vi "VariantToPlainText (Standard).vi"(11 "Variant-formatted Value":variant) -> (3 "String-formatted Value":string)   [LabVIEW 2013, in "OpenSerializer.lvlib" / "Serializer.PlainText.lvclass"]
uses:
  Serializer.PlainText.lvclass
  <vilib>/LabVIEW Open Source Project/Data Manipulation/TypeDescriptor/TypeDescriptor_GetName.vi
  <vilib>/LabVIEW Open Source Project/Data Manipulation/TypeDescriptor/TypeDescriptor_GetType.vi
  <vilib>/LabVIEW Open Source Project/Data Manipulation/TypeDescriptor/TypeDescriptor_GetPString.vi
  <vilib>/LabVIEW Open Source Project/Data Manipulation/Conversions/Flattened nD-Array to Flattened 1D-Array.vi
  <vilib>/Utility/VariantDataType/VariantType.lvlib
  <vilib>/LabVIEW Open Source Project/Data Manipulation/TypeDescriptor/OpenDescriptor.lvlib
  <vilib>/LabVIEW Open Source Project/Data Manipulation/Variant/OpenVariant.lvlib
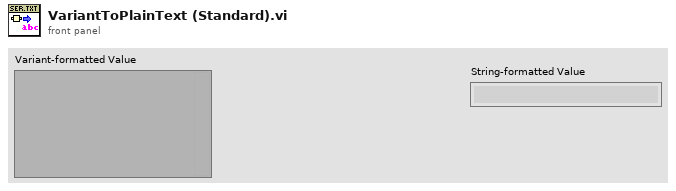
[diagram p1: front panel]
types:
  T1 = typedef "VariantType.lvlib/Type.ctl" = enum8{"Invalid Type", "Void", "I8", "I16", "I32", "I64", "U8", "U16", "U32", "U64", "Single Float", "Double Float", "Extended Float", "Single Complex", "Double Complex", "Extended Complex", "Enum U8", "Enum U16", "Enum U32", "Enum U64", "Single Float With Unit", "Double Float With Unit", "Extended Float With Unit", "Single Complex with Unit", "Double Complex with Unit", "Extended Complex with Unit", "Boolean", "String", "Path", "Picture", "Tag", "Array", "Cluster", "Variant", "LV Variant", "Waveform", "Timestamp", "Digital Waveform", "Digital Data", "ExpressData", "Refnum", "External Data", "VI", "Poly VI", "LabVIEW Class Instance", "Fixed Point"}
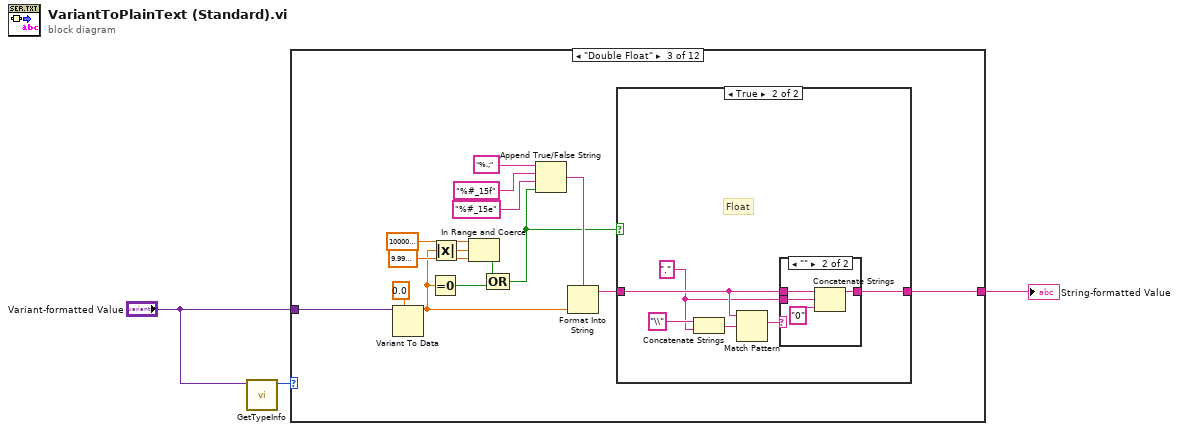
[diagram p0: block diagram]
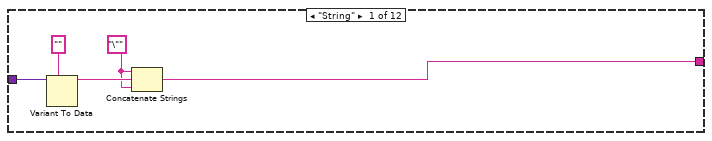
[diagram p2: hidden frame]
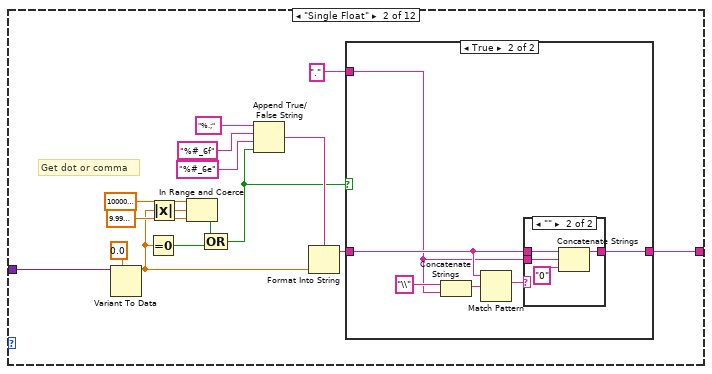
[diagram p3: hidden frame]
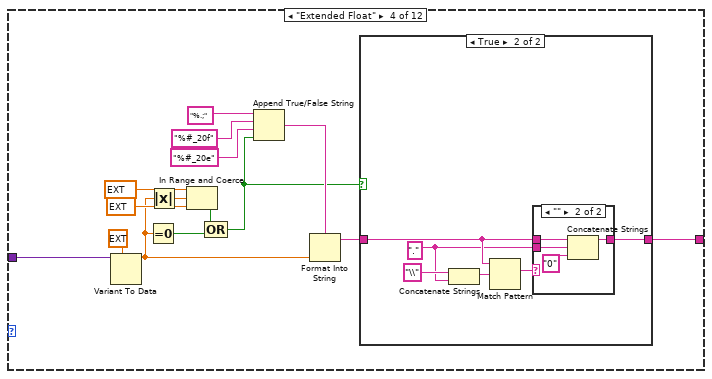
[diagram p8: hidden frame]
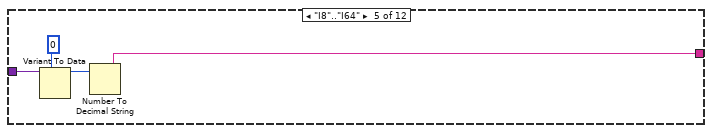
[diagram p11: hidden frame]
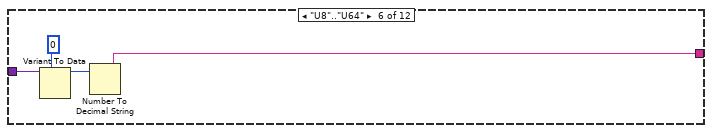
[diagram p12: hidden frame]
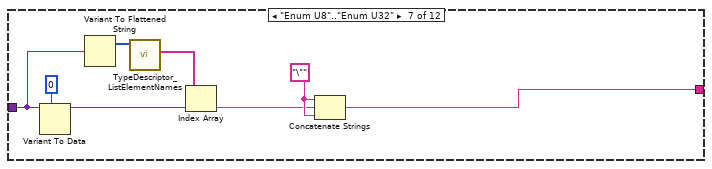
[diagram p13: hidden frame]
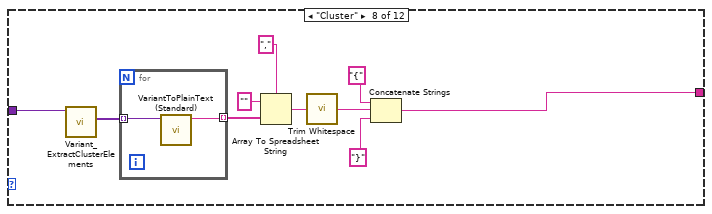
[diagram p14: hidden frame]
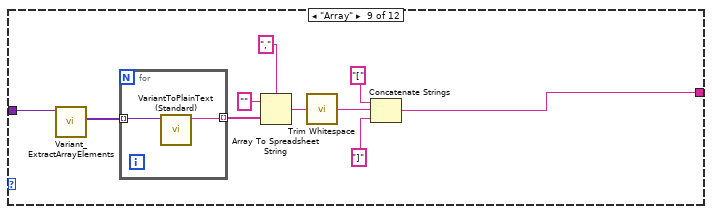
[diagram p15: hidden frame]
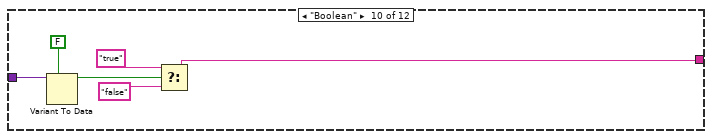
[diagram p16: hidden frame]
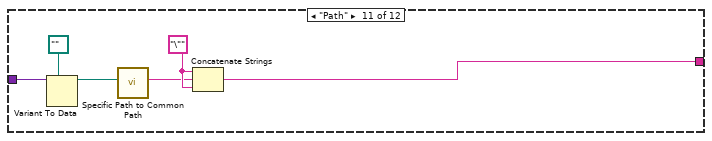
[diagram p17: hidden frame]
diagram:
  n1 = call <vilib>:"GetTypeInfo.vi"("Variant"="Variant-formatted Value") -> ("Type Enum"=w3:T1)  [unwired: 6 in, 4 out]
  n2 = case shown="\"Double Float\"" w3 {
    tunnel: "Variant-formatted Value" -> [w8 w18 w45 w72 w92 w96 w105 w113 w120 w136 w142 _]
    tunnel: [w5 w13 w40 w67 w91 w95 w99 w115 w127 w133 w139 _] -> w1
    frame "String" {
      w4 = "\"" ("Format String")
      n3 = Variant To Data(type="" ("Format String"), Variant=w8) -> (data=w6:string)  [unwired: 1 in, 1 out]
      n4 = Concatenate Strings(w4, w6, w4) -> (w5:string)
    }
    frame "Single Float" {
      # "Get dot or comma"
      n5 = Variant To Data(type=sgl 0.0, Variant=w18) -> (data=w15:sgl)  [unwired: 1 in, 1 out]
      n6 = Equal To 0?(x=w15) -> (x = 0?=w20:bool)
      n7 = Absolute Value(x=w15) -> (abs(x)=w21:sgl)
      n8 = In Range and Coerce(upper limit=sgl 1000000.0, x=w21, lower limit=sgl 0.0001 ("upper limit")) -> (In Range?=w19:bool)  [unwired: 1 out]
      n9 = Compound Arithmetic op=OR(w19, w20) -> (w11:bool)
      n10 = Append True/False String(1:w11, 2:"%#_6e" ("format string"), 3:"%#_6f" ("format string"), 4:"%.;" ("format string")) -> (0:w14:string)
      n11 = Format Into String(format string=w14, w15) -> (resulting string=w12:string)  [unwired: 2 in, 1 out]
      n12 = case shown="True" w11 {
        tunnel: [w25 w31] -> w13
        tunnel: w12 -> [w25 w29]
        tunnel: "." ("regular expression") -> [_ w27]
        frame False {
        }
        frame True {
          n13 = Concatenate Strings("\\" ("string"), w27) -> (w26:string)
          n14 = Match Pattern(string=w29, regular expression=w26) -> (match substring=w30:string)  [unwired: 1 in, 3 out]
          n15 = case shown="\"\"" w30 {
            tunnel: w29 -> [w32 w35]
            tunnel: [w32 w36] -> w31
            tunnel: w27 -> [_ w33]
            frame Default {
            }
            frame "" {
              n16 = Concatenate Strings(w35, w33, "0" ("regular expression")) -> (w36:string)
            }
          }
        }
      }
    }
    frame "Double Float" {
      n17 = Variant To Data(type=0.0, Variant=w45) -> (data=w42:dbl)  [unwired: 1 in, 1 out]
      n18 = Equal To 0?(x=w42) -> (x = 0?=w47:bool)
      n19 = Absolute Value(x=w42) -> (abs(x)=w48:dbl)
      n20 = In Range and Coerce(upper limit=1000000.0, x=w48, lower limit=9.999999747378752e-05 ("upper limit")) -> (In Range?=w46:bool)  [unwired: 1 out]
      n21 = Compound Arithmetic op=OR(w46, w47) -> (w38:bool)
      n22 = Append True/False String(1:w38, 2:"%#_15e" ("format string"), 3:"%#_15f" ("format string"), 4:"%.;" ("format string")) -> (0:w41:string)
      n23 = Format Into String(format string=w41, w42) -> (resulting string=w39:string)  [unwired: 2 in, 1 out]
      n24 = case shown="True" w38 {
        tunnel: [w52 w58] -> w40
        tunnel: w39 -> [w52 w56]
        frame False {
          # "Exponential"
        }
        frame True {
          w53 = "." ("regular expression")
          # "Float"
          n25 = Concatenate Strings("\\" ("string"), w53) -> (w54:string)
          n26 = Match Pattern(string=w56, regular expression=w54) -> (match substring=w57:string)  [unwired: 1 in, 3 out]
          n27 = case shown="\"\"" w57 {
            tunnel: w56 -> [w59 w62]
            tunnel: [w59 w63] -> w58
            tunnel: w53 -> [_ w60]
            frame Default {
            }
            frame "" {
              n28 = Concatenate Strings(w62, w60, "0" ("regular expression")) -> (w63:string)
            }
          }
        }
      }
    }
    frame "Extended Float" {
      n29 = Variant To Data(type=ext 0.0, Variant=w72) -> (data=w69:ext)  [unwired: 1 in, 1 out]
      n30 = Equal To 0?(x=w69) -> (x = 0?=w74:bool)
      n31 = Absolute Value(x=w69) -> (abs(x)=w75:ext)
      n32 = In Range and Coerce(upper limit=ext 1000000.0, x=w75, lower limit=ext 9.999999747378752e-05 ("upper limit")) -> (In Range?=w73:bool)  [unwired: 1 out]
      n33 = Compound Arithmetic op=OR(w73, w74) -> (w65:bool)
      n34 = Append True/False String(1:w65, 2:"%#_20e" ("format string"), 3:"%#_20f" ("format string"), 4:"%.;" ("format string")) -> (0:w68:string)
      n35 = Format Into String(format string=w68, w69) -> (resulting string=w66:string)  [unwired: 2 in, 1 out]
      n36 = case shown="True" w65 {
        tunnel: [w79 w85] -> w67
        tunnel: w66 -> [w79 w83]
        frame False {
        }
        frame True {
          w80 = "." ("regular expression")
          n37 = Concatenate Strings("\\" ("string"), w80) -> (w81:string)
          n38 = Match Pattern(string=w83, regular expression=w81) -> (match substring=w84:string)  [unwired: 1 in, 3 out]
          n39 = case shown="\"\"" w84 {
            tunnel: w83 -> [w86 w89]
            tunnel: [w86 w90] -> w85
            tunnel: w80 -> [_ w87]
            frame Default {
            }
            frame "" {
              n40 = Concatenate Strings(w89, w87, "0" ("regular expression")) -> (w90:string)
            }
          }
        }
      }
    }
    frame "I8".."I64" {
      n41 = Variant To Data(type=i64 0, Variant=w92) -> (data=w93:i64)  [unwired: 1 in, 1 out]
      n42 = Number To Decimal String(number=w93) -> (decimal integer string=w91:string)  [unwired: 1 in]
    }
    frame "U8".."U64" {
      n43 = Variant To Data(type=u64 0, Variant=w96) -> (data=w97:u64)  [unwired: 1 in, 1 out]
      n44 = Number To Decimal String(number=w97) -> (decimal integer string=w95:string)  [unwired: 1 in]
    }
    frame "Enum U8".."Enum U32" {
      w101 = "\"" ("Format String")
      n45 = Variant To Data(type=0, Variant=w105) -> (data=w102:i32)  [unwired: 1 in, 1 out]
      n46 = Variant To Flattened String(Variant=w105) -> (1:w104:i16[])  [unwired: 1 out]
      n47 = call <vilib>:"TypeDescriptor_ListElementNames.vi"("type descriptor"=w104) -> ("element names"=w103:string[])  [unwired: 7 in, 3 out]
      n48 = Index Array(array=w103, index=w102) -> (element=w100:string)
      n49 = Concatenate Strings(w101, w100, w101) -> (w99:string)
    }
    frame "Cluster" {
      n50 = call <vilib>:"Variant_ExtractClusterElements.vi"("Cluster"=w113) -> ("Elements"=w112:variant[])  [unwired: 8 in, 2 out]
      n51 = for {
        tunnel: w112 -> [w118] mode=indexing
        tunnel: [w117] -> w111 mode=indexing
        n52 = call "VariantToPlainText (Standard).vi"("Variant-formatted Value"=w118) -> ("String-formatted Value"=w117:string)  [unwired: 10 in]
      }
      n53 = Array To Spreadsheet String(delimiter (Tab)="," ("Format String"), array=w111, 3:"" ("format string")) -> (spreadsheet string=w108:string)
      n54 = call <vilib>:"Trim Whitespace.vi"("string"=w108) -> ("trimmed string"=w107:string)  [unwired: 1 in]
      n55 = Concatenate Strings("{" ("Format String"), w107, "}" ("Format String")) -> (w115:string)
    }
    frame "Array" {
      n56 = call <vilib>:"Variant_ExtractArrayElements.vi"("Array"=w120) -> ("Elements"=w119:variant[])  [unwired: 7 in, 3 out]
      n57 = for {
        tunnel: w119 -> [w130] mode=indexing
        tunnel: [w129] -> w125 mode=indexing
        n58 = call "VariantToPlainText (Standard).vi"("Variant-formatted Value"=w130) -> ("String-formatted Value"=w129:string)  [unwired: 10 in]
      }
      n59 = Array To Spreadsheet String(delimiter (Tab)="," ("Format String"), array=w125, 3:"" ("format string")) -> (spreadsheet string=w122:string)
      n60 = call <vilib>:"Trim Whitespace.vi"("string"=w122) -> ("trimmed string"=w121:string)  [unwired: 1 in]
      n61 = Concatenate Strings("[" ("Format String"), w121, "]" ("Format String")) -> (w127:string)
    }
    frame "Boolean" {
      n62 = Variant To Data(type=FALSE, Variant=w136) -> (data=w134:bool)  [unwired: 1 in, 1 out]
      n63 = Select(t="true", s=w134, f="false") -> (s? t:f=w133:string)
    }
    frame "Path" {
      w140 = "\"" ("Format String")
      n64 = Variant To Data(type=path "" ("Format String"), Variant=w142) -> (data=w138:path)  [unwired: 1 in, 1 out]
      n65 = call "Specific Path to Common Path.vi"("specific path"=w138) -> ("common path"=w137:string)  [unwired: 10 in]
      n66 = Concatenate Strings(w140, w137, w140) -> (w139:string)
    }
    frame Default {
    }
  }
  "String-formatted Value" <- w1
